vi "deleta trecho de onda.vi"(9 "Waveform":waveform(dbl), 11 "reference":refnum<vi>) -> (2 "New Waveform":waveform(dbl))   [LabVIEW 2019]
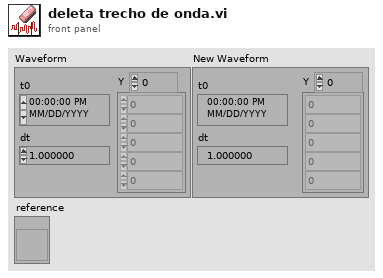
[diagram p1: front panel]
types:
  T1 = typedef "LVCursorListTypeDef.ctl" = cluster{"Name":string, "Color":u32, "Style":u8, "Point Style":u8, "Name Visible":bool, "Allow Drag":bool, "Cursor Mode":u32, "Plot":i32, "Index":i32, "Position":cluster{"X":dbl, "Y":dbl}, "X Scale":u32, "Y Scale":u32, "Watch Plots":i32[], "Watch All Plots":bool, "Plot Area":i32, "Label Offset":cluster{"X":dbl, "Y":dbl}}[]
  T2 = cluster{"Name":string, "Color":u32, "Style":u8, "Point Style":u8, "Name Visible":bool, "Allow Drag":bool, "Cursor Mode":u32, "Plot":i32, "Index":i32, "Position":cluster{"X":dbl, "Y":dbl}, "X Scale":u32, "Y Scale":u32, "Watch Plots":i32[], "Watch All Plots":bool, "Plot Area":i32, "Label Offset":cluster{"X":dbl, "Y":dbl}}
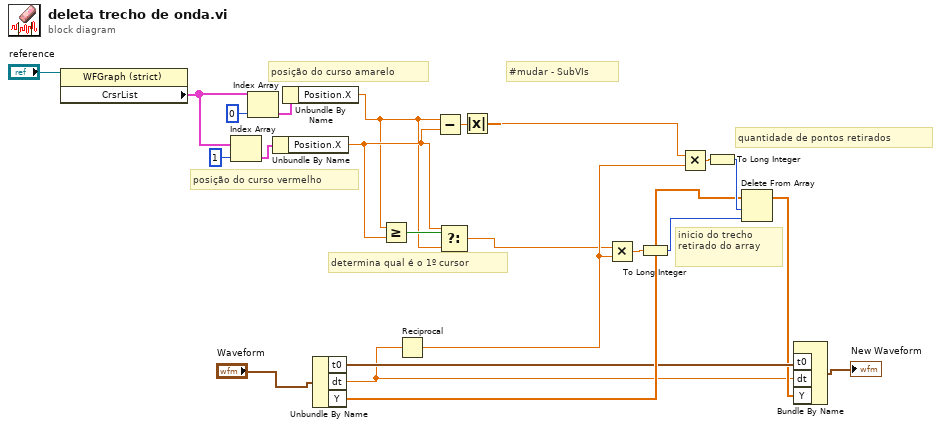
[diagram p0: block diagram]
diagram:
  # "#mudar - SubVIs"
  # "inicio do trecho\nretirado do array"
  # "determina qual é o 1º cursor"
  # "quantidade de pontos retirados"
  # "posição do curso vermelho"
  # "posição do curso amarelo"
  n1 = property on="Property Node" class="WFGraph (strict)"(reference="reference") -> ("CrsrList"=w20:T1)  [unwired: 1 in, 2 out]
  n2 = Index Array(array=w20, index=1) -> (element=w19:T2)
  n3 = Index Array(array=w20, index=0) -> (element=w22:T2)
  n4 = Unbundle By Name(w19) -> ("Position.X"=w6:dbl)
  n5 = Unbundle By Name(w22) -> ("Position.X"=w4:dbl)
  n6 = Unbundle By Name("Waveform") -> ("t0"=w15:timestamp, "dt"=w13:dbl, "Y"=w16:dbl[])
  n7 = Greater Or Equal?(x=w4, y=w6) -> (x >= y?=w7:bool)
  n8 = Reciprocal(x=w13) -> (1/x=w12:dbl)
  n9 = Subtract(x=w4, y=w6) -> (x-y=w9:dbl)
  n10 = Select(t=w6, s=w7, f=w4) -> (s? t:f=w5:dbl)
  n11 = Absolute Value(x=w9) -> (abs(x)=w8:dbl)
  n12 = Multiply(x=w5, y=w12) -> (x*y=w11:dbl)
  n13 = To Long Integer(number=w11) -> (32bit integer=w10:i32)
  n14 = Multiply(x=w8, y=w12) -> (x*y=w18:dbl)
  n15 = To Long Integer(number=w18) -> (32bit integer=w17:i32)
  n16 = Delete From Array(array=w16, length=w17, index=w10) -> (array with subset deleted=w14:dbl[])  [unwired: 1 out]
  n17 = Bundle By Name("t0"=w15, "dt"=w13, "Y"=w14) -> (→"New Waveform":waveform(dbl))  [unwired: 1 in]
